vi "libssh2_agent_connect.vi"(8 "error in (no error)":errorcluster, 11 "agent":T1) -> (0 "error out":errorcluster)   [LabVIEW 2013, in "libssh2.lvlib"]
doc: "Connects to the ssh agent."
uses:
  libssh2.lvlib
  Agent Refnum.ctl
  Global Settings.vi
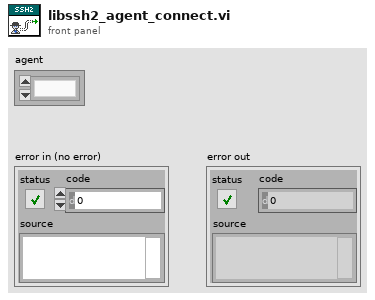
[diagram p1: front panel]
types:
  T1 = typedef "libssh2.lvlib/Agent Refnum.ctl" = refnum<k1>
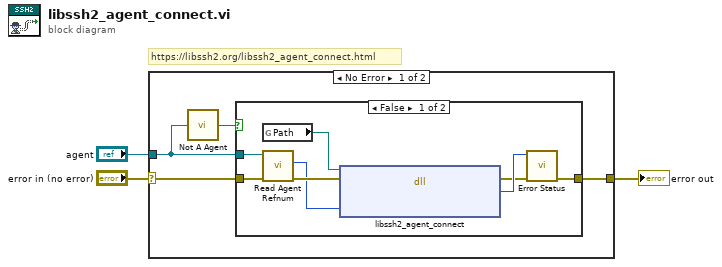
[diagram p0: block diagram]
diagram:
  # "https://libssh2.org/libssh2_agent_connect.html"
  n1 = case shown="No Error" "error in (no error)" {
    selector: "error in (no error)" -> [w6 w17]
    tunnel: [w7 w17] -> w3
    tunnel: "agent" -> [w5 _]
    frame No Error {
      n2 = call "Not A Agent.vi"("agent"=w5) -> ("Not a Agent?"=w4:bool)
      n3 = case shown="False" w4 {
        tunnel: [w13 w16] -> w7
        tunnel: w6 -> [w11 w16]
        tunnel: w5 -> [w8 _]
        frame False {
          n4 = global read "Global Settings.vi" "Path"() -> (w12:path)
          n5 = call "Read Agent Refnum.vi"("error in (no error)"=w11, "agent"=w8) -> ("error out"=w10:errorcluster, "LIBSSH2_AGENT*"=w9:u64)  [unwired: 8 in]
          n6 = dll-call lib="C:/Users/pasca/source/repos/libssh2-labview/libssh2/libssh2**.*" fn="libssh2_agent_connect"(path in=w12, error in=w10, "agent"=w9) -> (error out=w14:errorcluster, "return value"=w15:i32)  [unwired: 2 in, 1 out]
          n7 = call "Error Status.vi"("error in (no error)"=w14, "return value"=w15) -> ("error out"=w13:errorcluster)  [unwired: 8 in, 1 out]
        }
        frame True {
        }
      }
    }
    frame Error {
    }
  }
  "error out" <- w3
